vi "Main.vi"() -> ()   [LabVIEW 2017, in "SSH.lvlib"]
doc: "This template is based off of the Queued Message Handler design pattern and the Queued Message Handler project template that ships with LabVIEW.\n\nThe main difference is that the queue is private to this module and communication between modules is performed via Broadcast and Request events.\n\nRequest events are wrapped in public API methods and are handled in the Event Handling Loop (EHL) of this VI. Any module can register for Broadcast events sent by this module. The EHL generates messages based on user interface actions.\n\nThe Message Handling Loop (MHL) processes messages generated by the EHL, or by other messages. The messages are string values, so new messages can be added easily to the Message Cases case structure in the MHL. Each message cluster can also provide an optional value for Message Data, which is a variant that can be converted to whatever message-specific data is required.\n_____\nBased on Delacor QMH Project Template 4.2.1.64."
uses:
  SSH.lvlib
  <vilib>/Delacor/Delacor QMH/Libraries/Cloneable Module Admin_class/Delacor_lib_QMH_Cloneable Module Admin.lvclass
  C:/Program Files (x86)/National Instruments/LabVIEW 2017/vi.lib/Delacor/Delacor QMH/Libraries/Module Admin_class/Delacor_lib_QMH_Module Admin.lvclass
  Connection Info.ctl
  Response Configuration.ctl
  Return Request Configuration.ctl
  Module Data--cluster.ctl
  <vilib>/Delacor/Delacor QMH/Libraries/Cloneable Module Admin_class/Delacor_lib_QMH_Cloneable Module Admin.lvclass/Delacor_lib_QMH_Cloneable Module Admin.ctl
  <vilib>/Delacor/Delacor QMH/Libraries/Message Queue_class/Delacor_lib_QMH_Message Queue.lvclass/Delacor_lib_QMH_Message Queue.ctl
  Stop Argument--cluster.ctl
  <vilib>/Delacor/Delacor QMH/Libraries/Module Admin_class/Delacor_lib_QMH_Module Admin.lvclass/Delacor_lib_QMH_Module Admin.ctl
  Write Command Argument--cluster.ctl
  Write Command (Reply Payload)--cluster.ctl
  Set Response Configuration Argument--cluster.ctl
  <vilib>/Delacor/Delacor QMH/Libraries/Cloneable Module Admin_class/Delacor_lib_QMH_Get Module ID.vi
  <vilib>/Delacor/Delacor QMH/Libraries/Message Queue_class/Delacor_lib_QMH_Enqueue Message (Single).vi
  <vilib>/Delacor/Delacor QMH/Libraries/Module Admin_class/Delacor_lib_QMH_Get External Launch.vi
  <vilib>/Utility/error.llb/Error Cluster From Error Code.vi
  C:/Users/ukhornp/Documents/SSH/References/Renci.SshNet.dll
  References/Renci.SshNet.dll
  <vilib>/ErrorRing/Error Ring.xnode
  <vilib>/Delacor/Delacor QMH/Libraries/Message Queue_class/Delacor_lib_QMH_Message Queue.lvclass
  Clone Registration/Clone Registration.lvlib
panel:
  in  "Response Configuration":T1
  out "Output":string
  out "Return Payload":string
  in  "Command":string
  in  "Connection Info":T2={"host IP"="", "port"=22, "username"="lanforge", "password"="lanforge", "Connection Name"=""}
  in  "Simulate MHL Error":bool
  in  "Simulate EHL Error":bool
  out "error out":errorcluster
  in  "Module Admin":refnum<class "Delacor_lib_QMH_Cloneable Module Admin.lvclass">
  out "Status":string
  # "Other QMH Modules communicate with this Module via its Public API (wrappers for its Request Events).\n\nThis Module communicates with other Modules via its Broadcast Events.\nAny module that wants to get these messages, just registers for this module's Broadcast events."
  # "This template is for the Delacor Modified Queued Message Handler design pattern.\n\nSee the block diagram for more information on how to use this template."
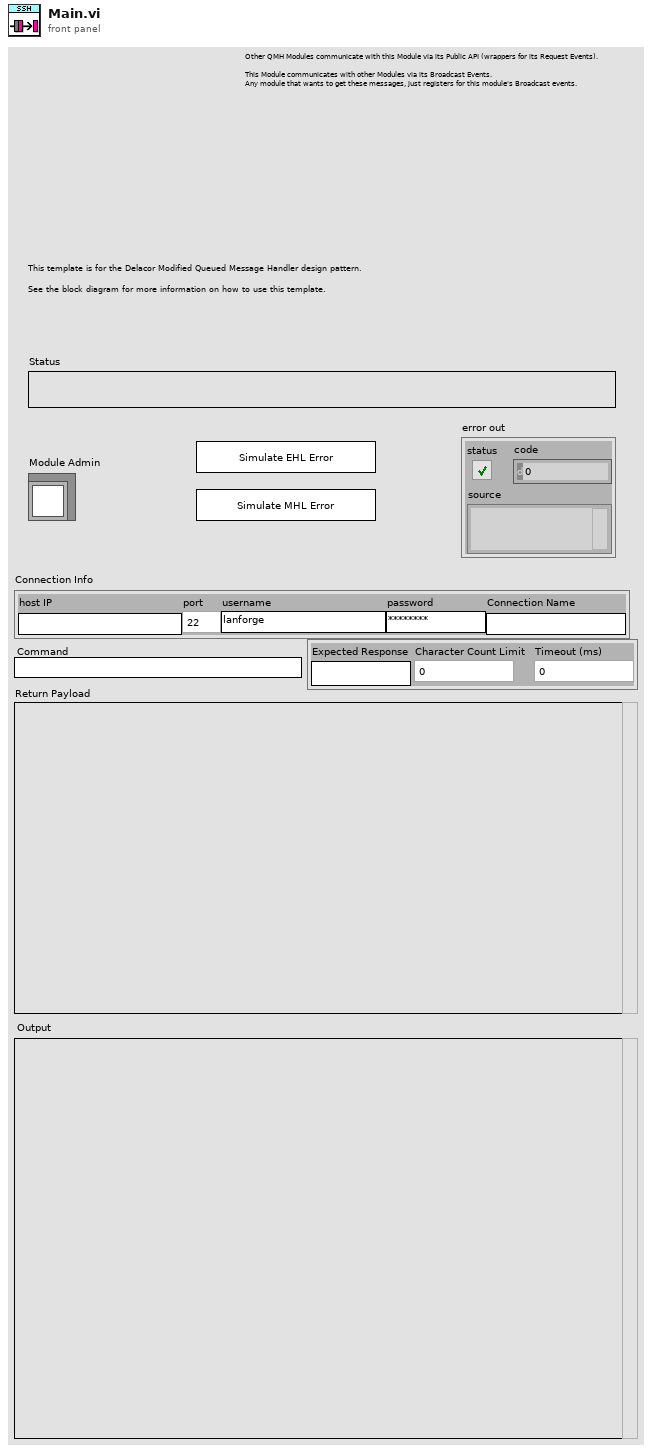
[diagram p1: front panel]
types:
  T1 = typedef "SSH.lvlib/Response Configuration.ctl" = cluster{"Expected Response":string, "Character Count Limit":i32, "Timeout (ms)":u32}
  T2 = typedef "SSH.lvlib/Connection Info.ctl" = cluster{"host IP":string, "port":i32, "username":string, "password":string, "Connection Name":string}
  T3 = typedef "SSH.lvlib/Return Request Configuration.ctl" = cluster{"Response Configuration":T1, "Return Notifier":refnum<notifier>, "Response Requested":bool, "Command":string, "Initial Timer Value":u32}
  T4 = typedef "SSH.lvlib/Request Events--cluster.ctl" = cluster{"Stop Module":refnum<user-event>, "Show Panel":refnum<user-event>, "Hide Panel":refnum<user-event>, "Show Diagram":refnum<user-event>, "Get Module Execution Status":refnum<user-event>, "Write Command":refnum<user-event>, "Set Response Configuration":refnum<user-event>}
  T5 = typedef "SSH.lvlib/Module Data--cluster.ctl" = cluster{"Status":string, "SSH Client Reference":refnum<k24>, "Shell Stream Reference":refnum<k24>, "Stream Writer Reference":refnum<k24>, "Response Configuration":T1}
  T6 = enum32{"invalid lock state", "Not Locked", "Locked (No Password)", "Password-protected"}
  T7 = typedef "SSH.lvlib/Stop Argument--cluster.ctl" = cluster{"Module ID":i32, "Origin":string, "Exit via Stop Module Req?":bool, "Wait for Module to stop?":bool}
  T8 = typedef "SSH.lvlib/Write Command Argument--cluster.ctl" = cluster{"Module ID":i32, "Command":string, "Wait Notifier":refnum<notifier>, "wait for reply":bool}
  T9 = typedef "SSH.lvlib/Set Response Configuration Argument--cluster.ctl" = cluster{"Module ID":i32, "Response Configuration":T1}
  T10 = enum32{"Invalid", "Standard", "Closed", "Hidden", "Minimized", "Maximized"}
  T11 = typedef "SSH.lvlib/dotNET references.ctl" = cluster{"SSH Client Reference":refnum<k24>, "Shell Stream Reference":refnum<k24>}
  T12 = typedef "eventvkey.ctl" = enum16{"ASCII", "Enter", "Return", "Shift", "Ctrl", "Alt", "Cmd", "Opt", "Caps", "NumLock", "Clear", "Break", "Up", "Down", "Left", "Right", "Insert", "Delete", "Home", "End", "PageUp", "PageDown", "Escape", "Help", "Pause", "ScrollLock", "F1", "F2", "F3", "F4", "F5", "F6", "F7", "F8", "F9", "F10", "F11", "F12", "F13", "F14", "F15", "F16", "F17", "F18", "F19", "F20", "F21", "F22", "F23", "F24", "Play", "VolumeUp", "VolumeDown", "Mute", "Two Byte Char"}
  T13 = typedef "SSH.lvlib/Write Command (Reply Payload)--cluster.ctl" = cluster{"Write Command_error":errorcluster, "Return String Payload":string}
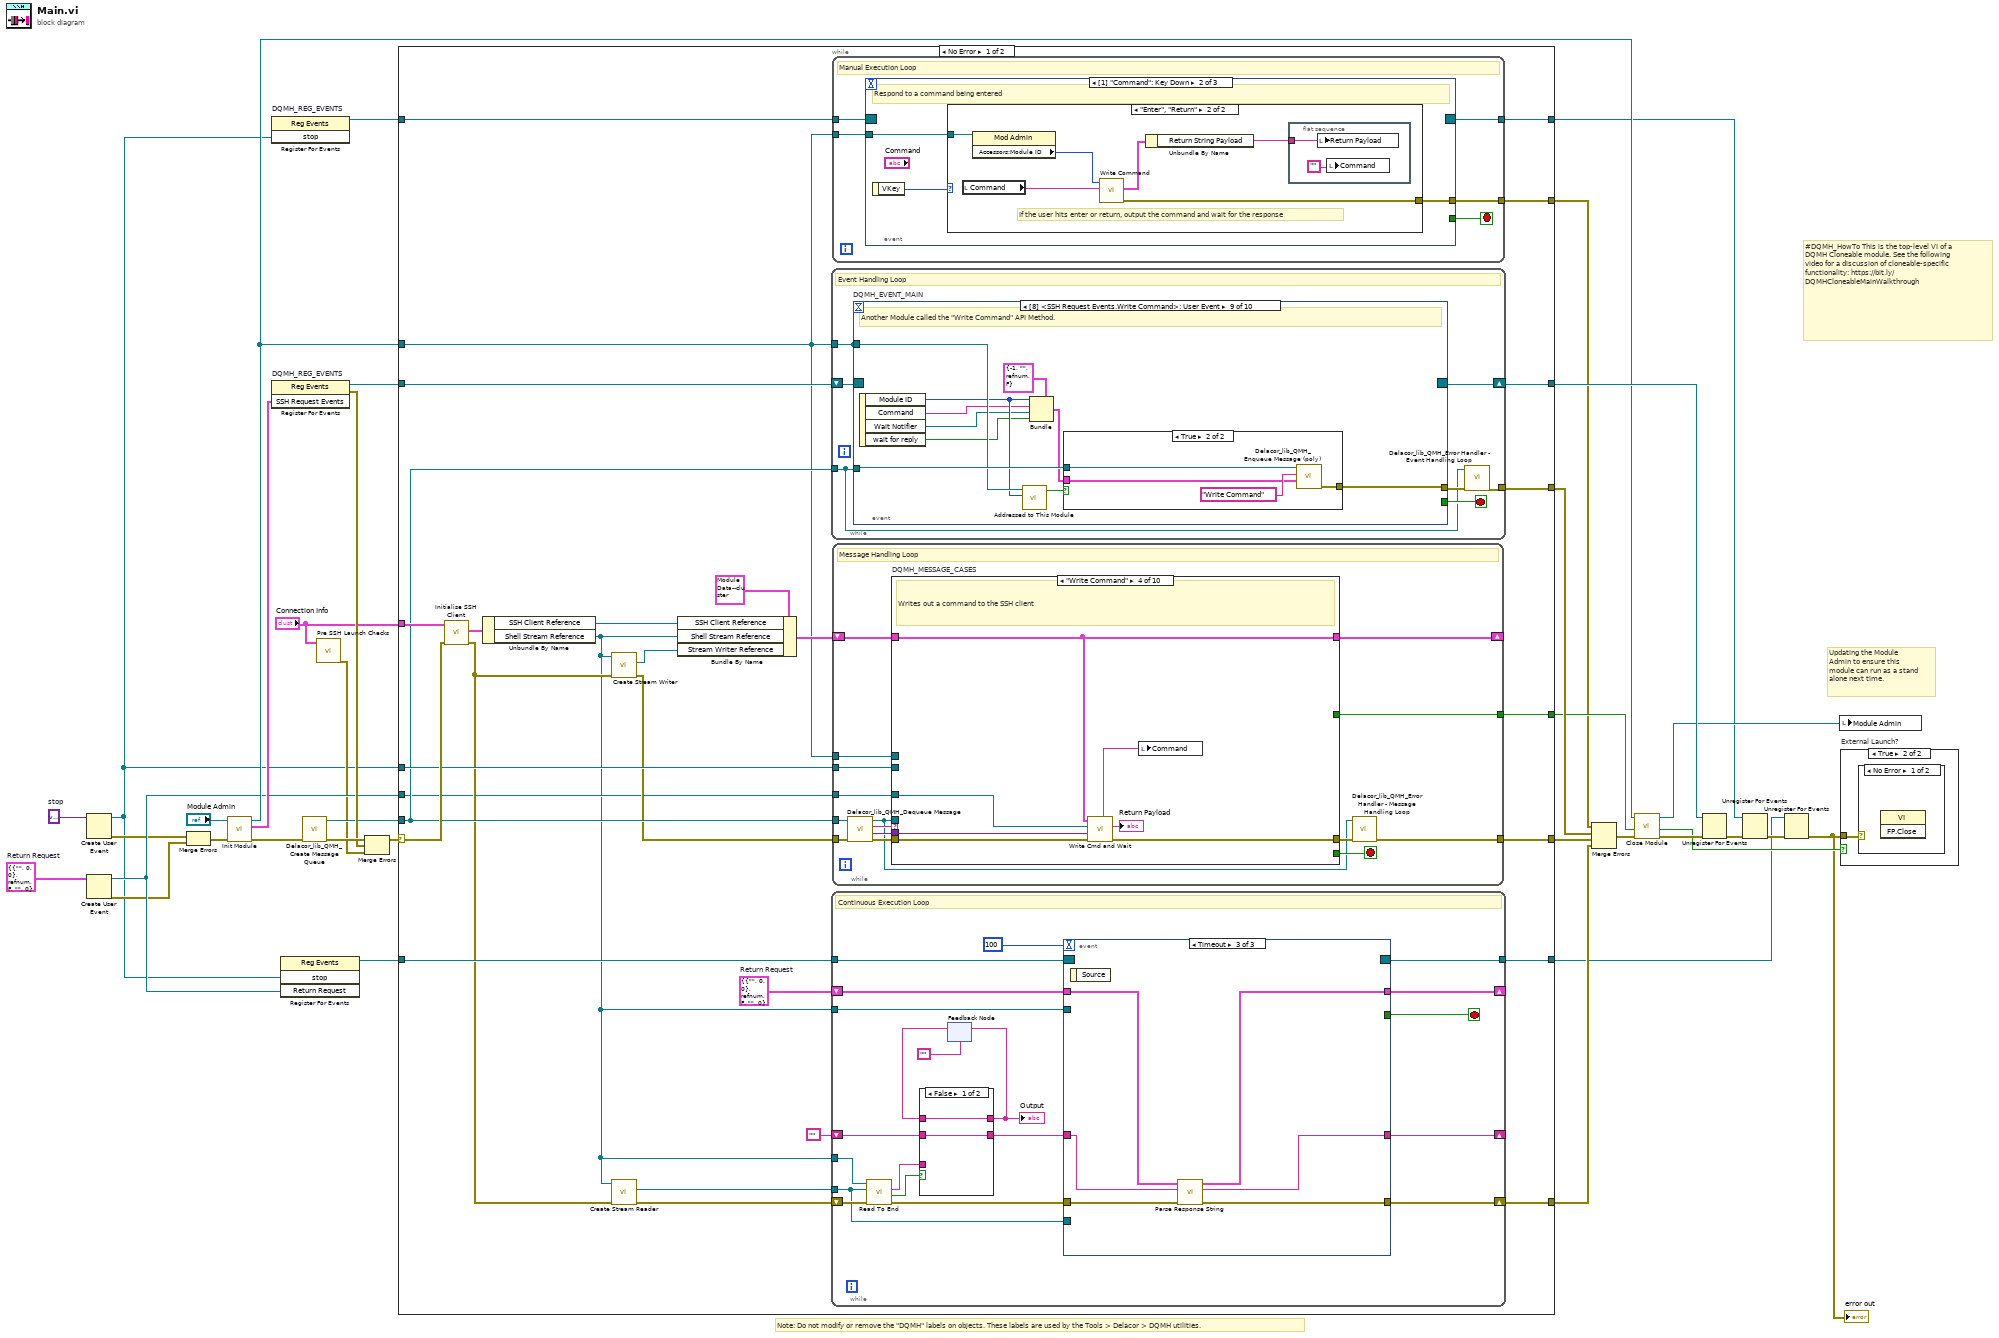
[diagram p0: block diagram]
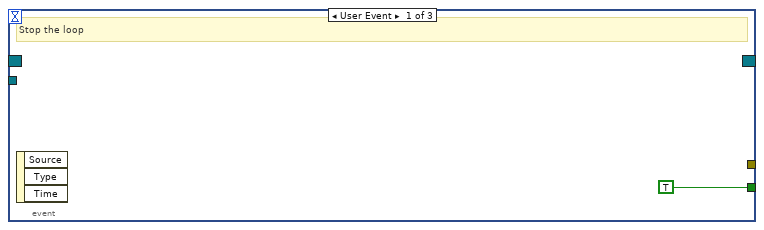
[diagram p2: hidden frame]
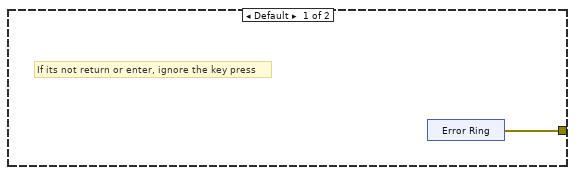
[diagram p3: hidden frame]
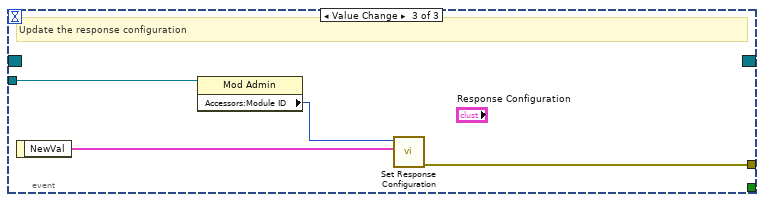
[diagram p4: hidden frame]
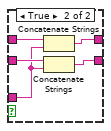
[diagram p5: hidden frame]
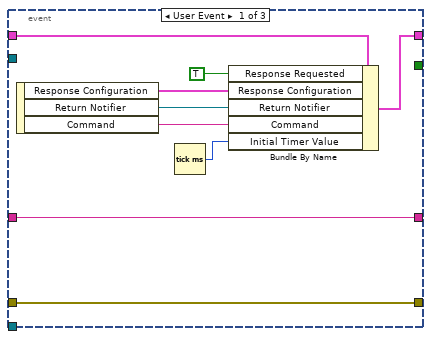
[diagram p6: hidden frame]
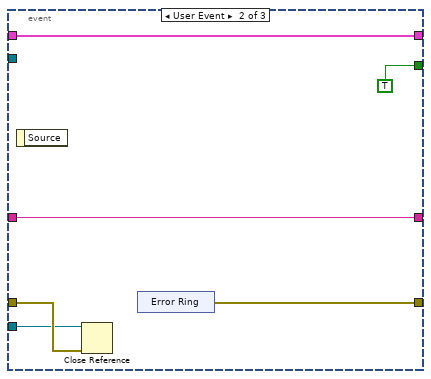
[diagram p7: hidden frame]
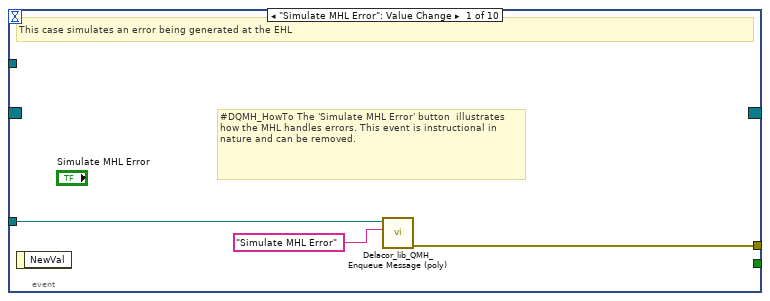
[diagram p8: hidden frame]
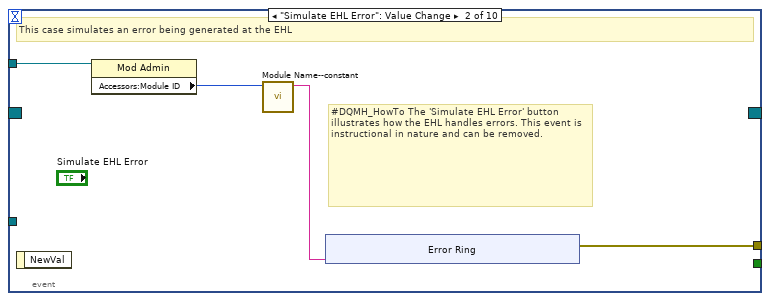
[diagram p9: hidden frame]
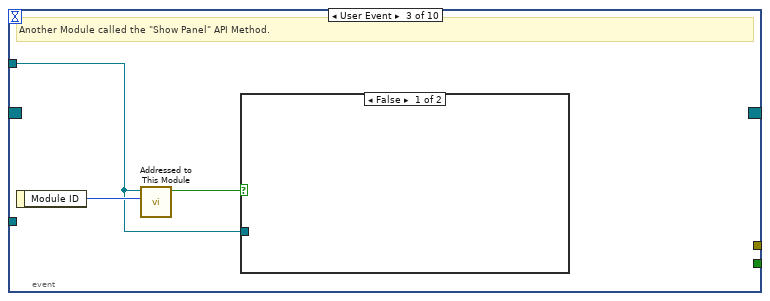
[diagram p10: hidden frame]
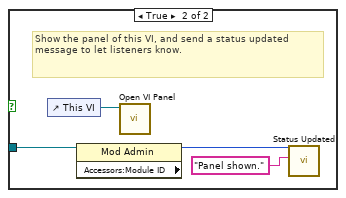
[diagram p11: hidden frame]
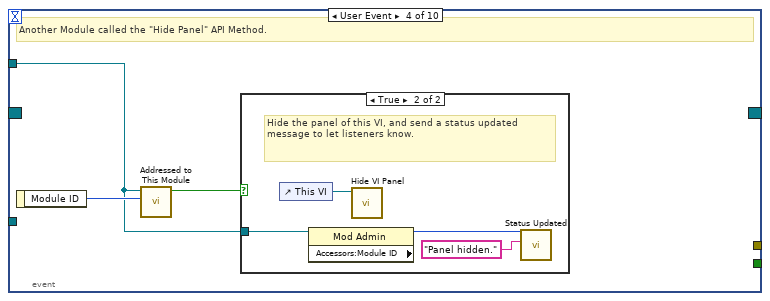
[diagram p12: hidden frame]
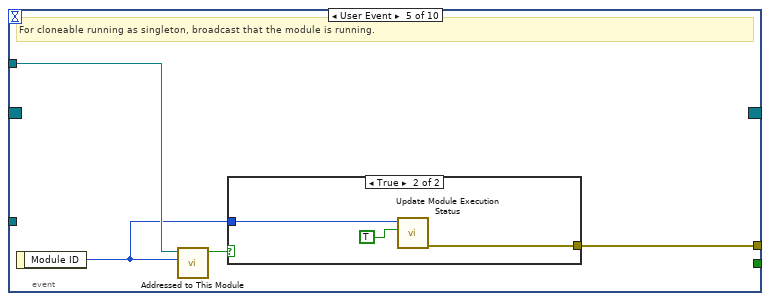
[diagram p14: hidden frame]
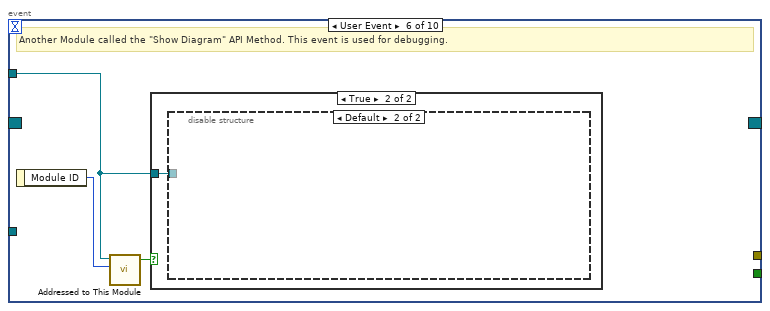
[diagram p16: hidden frame]
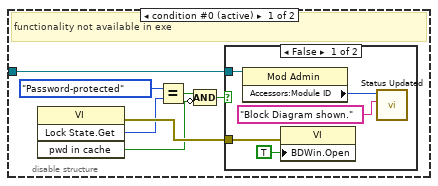
[diagram p18: hidden frame]
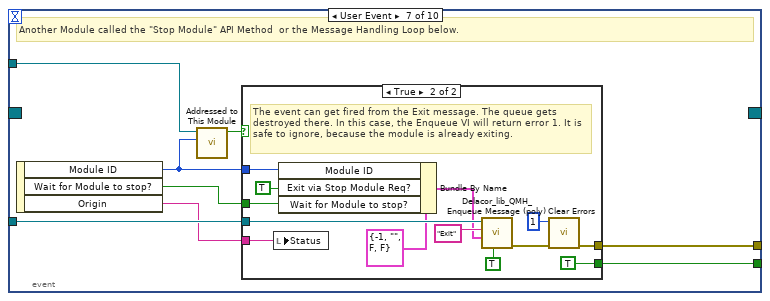
[diagram p20: hidden frame]
diagram:
  w14 = T3 {"Response Configuration"={"Expected Response"="", "Character Count Limit"=0, "Timeout (ms)"=0}, "Return Notifier"=refnum, "Response Requested"=FALSE, "Command"="", "Initial Timer Value"=0}  # Return Request
  w17 = variant  # stop
  # "#DQMH_HowTo This is the top-level VI of a DQMH Cloneable module. See the following video for a discussion of cloneable-specific functionality: https://bit.ly/DQMHCloneableMainWalkthrough"
  # "Note: Do not modify or remove the \"DQMH\" labels on objects. These labels are used by the Tools > Delacor > DQMH utilities."
  # "Updating the Module Admin to ensure this module can run as a stand alone next time."
  n1 = Create User Event(user event datatype=w17) -> (user event=w5:refnum<user-event>, error out=w10:errorcluster)  [unwired: 1 in]
  n2 = Create User Event(user event datatype=w14) -> (user event=w13:refnum<user-event>, error out=w11:errorcluster)  [unwired: 1 in]
  n3 = Merge Errors(w10, w11) -> (w9:errorcluster)
  n4 = call "Init Module.vi"("error in (no error)"=w9, "Cloneable Module Admin in"="Module Admin") -> ("error out"=w32:errorcluster, "SSH Request Events"=w24:T4, "Cloneable Module Admin out"=w21:refnum<class "Delacor_lib_QMH_Cloneable Module Admin.lvclass">)  [unwired: 7 in]
  n5 = register-events "DQMH_REG_EVENTS"(w5) -> (reference out=w6:refnum<event-registration>)  [unwired: 2 in, 1 out]
  n6 = register-events "DQMH_REG_EVENTS"(w24) -> (reference out=w25:refnum<event-registration>, error out=w27:errorcluster)  [unwired: 2 in]
  n7 = register-events(w5, w13) -> (reference out=w16:refnum<event-registration>)  [unwired: 2 in, 1 out]
  n8 = call <vilib>:"Delacor_lib_QMH_Create Message Queue.vi"("error in (no error)"=w32) -> ("error out"=w29:errorcluster, "Message Queue"=w23:refnum<class "Delacor_lib_QMH_Message Queue.lvclass">)  [unwired: 9 in]
  n9 = call "Pre SSH Launch Checks.vi"("Connection Info"="Connection Info") -> ("error out"=w7:errorcluster)  [unwired: 10 in]
  n10 = Merge Errors(w29, w27, w7) -> (w28:errorcluster)
  n11 = case shown="No Error" w28 {
    selector: w28 -> [w57 w387]
    tunnel: [w64 w387] -> w33
    tunnel: [w62 w386] -> w26
    tunnel: w25 -> [w60 w386]
    tunnel: w23 -> [w50 _]
    tunnel: [w63 _] -> w34
    tunnel: w21 -> [w38 w382]
    tunnel: [w59 _] -> w19
    tunnel: "Connection Info" -> [w56 _]
    tunnel: [w53 w379] -> w1
    tunnel: w16 -> [w52 w379]
    tunnel: w5 -> [w51 _]
    tunnel: w13 -> [w44 _]
    tunnel: [w43 _] -> w12
    tunnel: w6 -> [w39 w378]
    tunnel: [w37 _] -> w4
    tunnel: [w36 w378] -> w2
    frame No Error {
      w42 = T3 {"Response Configuration"={"Expected Response"="", "Character Count Limit"=0, "Timeout (ms)"=0}, "Return Notifier"=refnum, "Response Requested"=FALSE, "Command"="", "Initial Timer Value"=0}  # Return Request
      n12 = call "Initialise SSH Client.vi"("error in (no error)"=w57, "Connection Info"=w56) -> ("error out"=w47:errorcluster, "References"=w55:T11)  [unwired: 8 in]
      n13 = Unbundle By Name(w55) -> ("SSH Client Reference"=w54:refnum<k24>, "Shell Stream Reference"=w41:refnum<k24>)
      n14 = call "Create Stream Writer.vi"("error in (no error)"=w47, "Shell Stream Ref"=w41) -> ("error out"=w48:errorcluster, "Stream Writer ref"=w49:refnum<k24>)  [unwired: 8 in]
      n15 = call "Create Stream Reader.vi"("error in (no error)"=w47, "Shell Stream Ref"=w41) -> ("error out"=w46:errorcluster, "Stream Reader Ref"=w45:refnum<k24>)  [unwired: 8 in]
      n16 = Bundle By Name(cluster=T5 {"Status"="", "SSH Client Reference"=refnum, "Shell Stream Reference"=refnum, "Stream Writer Reference"=refnum, "Response Configuration"={"Expected Response"="", "Character Count Limit"=0, "Timeout (ms)"=0}} ("Data Cluster"), "SSH Client Reference"=w54, "Shell Stream Reference"=w41, "Stream Writer Reference"=w49) -> (w58:T5)
      n17 = while {
        tunnel: w50 -> [w138]
        shift-right: [w140] -> w62
        shift-left: w60 -> [w141]
        tunnel: [w142] -> w63
        tunnel: w38 -> [w137]
        tunnel: [w137] -> _
        stop <- w139 stop-if-true
        # "Event Handling Loop"
        n18 = event "DQMH_EVENT_MAIN" shown="[8] <SSH Request Events.Write Command>: User Event" {
          selector: w141 -> [_ _ _ _ _ _ _ _ _ _]
          dyn-events: [_ _ _ _ _ _ _ _ _ _] -> w140
          timeout: _ -> [_ _ _ _ _ _ _ _ _ _]
          tunnel: [_ _ _ _ _ _ w198 _ _ _] -> w139
          tunnel: w138 -> [w145 _ _ _ _ _ w201 w217 w235 w247]
          tunnel: [w146 w150 _ _ w175 _ w202 w220 w228 w240] -> w143
          tunnel: w137 -> [_ w149 w158 w165 w173 w179 w200 w218 w233 w245]
          event "Simulate MHL Error": Value Change {
            # "#DQMH_HowTo The 'Simulate MHL Error' button  illustrates how the MHL handles errors. This event is instructional in nature and can be removed."
            # "This case simulates an error being generated at the EHL"
            n19 = event-data() -> ()  [unwired: 1 in, 1 out]
            n20 = call-poly <vilib>:"Delacor_lib_QMH_Enqueue Message (poly).vi"("Message"="Simulate MHL Error", "Message Queue in"=w145) -> ("error out"=w146:errorcluster)  [unwired: 8 in, 1 out]
          }
          event "Simulate EHL Error": Value Change {
            # "#DQMH_HowTo The 'Simulate EHL Error' button  illustrates how the EHL handles errors. This event is instructional in nature and can be removed."
            # "This case simulates an error being generated at the EHL"
            n21 = event-data() -> ()  [unwired: 1 in, 1 out]
            n22 = property class="Mod Admin"(reference=w149) -> ("Accessors:Module ID"=w148:i32)  [unwired: 1 in, 2 out]
            n23 = call "Module Name--constant.vi"("Module ID"=w148) -> ("Module Name"=w147:string)  [unwired: 10 in]
            n24 = xnode "Error Ring"("parameter 0"=w147) -> ("error out"=w150:errorcluster)
          }
          event User Event {
            # "Another Module called the \"Show Panel\" API Method."
            n25 = event-data() -> ("Module ID"=w159:i32)  [unwired: 1 in]
            n26 = call "Addressed to This Module.vi"("Module ID from Argument"=w159, "Module Admin"=w158) -> ("Addressed to this instance?"=w160:bool)  [unwired: 8 in, 1 out]
            n27 = case shown="False" w160 {
              tunnel: w158 -> [_ w162]
              frame False {
              }
              frame True {
                # "Show the panel of this VI, and send a status updated message to let listeners know."
                n28 = control-ref of="This VI"() -> (w164:refnum<vi>)
                n29 = property class="Mod Admin"(reference=w162) -> ("Accessors:Module ID"=w161:i32)  [unwired: 1 in, 2 out]
                n30 = call "Open VI Panel.vi"("VI"=w164) -> ()  [unwired: 10 in, 1 out]
                n31 = call "Status Updated.vi"("Status"="Panel shown." ("format string"), "Module ID"=w161) -> ()  [unwired: 9 in, 1 out]
              }
            }
          }
          event User Event {
            # "Another Module called the \"Hide Panel\" API Method."
            n32 = event-data() -> ("Module ID"=w166:i32)  [unwired: 1 in]
            n33 = call "Addressed to This Module.vi"("Module ID from Argument"=w166, "Module Admin"=w165) -> ("Addressed to this instance?"=w167:bool)  [unwired: 8 in, 1 out]
            n34 = case shown="True" w167 {
              tunnel: w165 -> [_ w169]
              frame False {
              }
              frame True {
                # "Hide the panel of this VI, and send a status updated message to let listeners know."
                n35 = control-ref of="This VI"() -> (w171:refnum<vi>)
                n36 = property class="Mod Admin"(reference=w169) -> ("Accessors:Module ID"=w168:i32)  [unwired: 1 in, 2 out]
                n37 = call "Hide VI Panel.vi"("VI"=w171) -> ()  [unwired: 10 in, 1 out]
                n38 = call "Status Updated.vi"("Status"="Panel hidden." ("format string"), "Module ID"=w168) -> ()  [unwired: 9 in, 1 out]
              }
            }
          }
          event User Event {
            # "For cloneable running as singleton, broadcast that the module is running."
            n39 = event-data() -> ("Module ID"=w172:i32)  [unwired: 1 in]
            n40 = call "Addressed to This Module.vi"("Module ID from Argument"=w172, "Module Admin"=w173) -> ("Addressed to this instance?"=w174:bool)  [unwired: 8 in, 1 out]
            n41 = case shown="True" w174 {
              tunnel: [_ w178] -> w175
              tunnel: w172 -> [_ w177]
              frame False {
              }
              frame True {
                n42 = call "Update Module Execution Status.vi"("Running?"=TRUE, "Module ID"=w177) -> ("error out"=w178:errorcluster)  [unwired: 9 in]
              }
            }
          }
          event User Event {
            # "Another Module called the \"Show Diagram\" API Method. This event is used for debugging."
            n43 = event-data() -> ("Module ID"=w180:i32)  [unwired: 1 in]
            n44 = call "Addressed to This Module.vi"("Module ID from Argument"=w180, "Module Admin"=w179) -> ("Addressed to this instance?"=w181:bool)  [unwired: 8 in, 1 out]
            n45 = case shown="True" w181 {
              tunnel: w179 -> [_ w182]
              frame False {
              }
              frame True {
                n46 = disable-structure shown="Default" {
                  disable-tunnel: w182 -> [w183 _]
                  frame condition #0 (active) {
                    # "functionality not available in exe"
                    n47 = invoke class="VI" method="Lock State.Get"() -> (error out=w189:errorcluster, "Get Lock State"=w188:T6, "pwd in cache"=w185:bool)  [unwired: 4 in, 1 out]
                    n48 = Equal?(x=T6."Password-protected", y=w188) -> (x = y?=w186:bool)
                    n49 = Compound Arithmetic op=AND(w186, invert w185) -> (w184:bool)
                    n50 = case shown="False" w184 {
                      tunnel: w189 -> [w194 _]
                      tunnel: w183 -> [w191 _]
                      frame False {
                        n51 = property class="Mod Admin"(reference=w191) -> ("Accessors:Module ID"=w190:i32)  [unwired: 1 in, 2 out]
                        n52 = property class="VI"(error in=w194, "BDWin.Open"=TRUE ("Block Diagram Window:Open")) -> ()  [unwired: 1 in, 2 out]
                        n53 = call "Status Updated.vi"("Status"="Block Diagram shown." ("format string"), "Module ID"=w190) -> ()  [unwired: 9 in, 1 out]
                      }
                      frame True {
                        # "Password-protected VI, and the password is not in the cache. Do not show the diagram."
                      }
                    }
                  }
                  frame condition #1 {
                  }
                }
              }
            }
          }
          event User Event {
            # "Another Module called the \"Stop Module\" API Method  or the Message Handling Loop below."
            n54 = event-data() -> ("Module ID"=w196:i32, "Wait for Module to stop?"=w197:bool, "Origin"=w195:string)  [unwired: 1 in]
            n55 = call "Addressed to This Module.vi"("Module ID from Argument"=w196, "Module Admin"=w200) -> ("Addressed to this instance?"=w199:bool)  [unwired: 8 in, 1 out]
            n56 = case shown="True" w199 {
              tunnel: [_ w214] -> w202
              tunnel: w201 -> [_ w210]
              tunnel: [_ TRUE] -> w198
              tunnel: w197 -> [_ w205]
              tunnel: w196 -> [_ w207]
              tunnel: w195 -> [_ w203]
              frame False {
              }
              frame True {
                # "The event can get fired from the Exit message. The queue gets destroyed there. In this case, the Enqueue VI will return error 1. It is safe to ignore, because the module is already exiting."
                n57 = local write "Status"(w203) -> ()
                n58 = Bundle By Name(cluster=T7 {"Module ID"=-1, "Origin"="", "Exit via Stop Module Req?"=FALSE, "Wait for Module to stop?"=FALSE} ("Stop Argument"), "Module ID"=w207, "Exit via Stop Module Req?"=TRUE, "Wait for Module to stop?"=w205) -> (w204:T7)
                n59 = call-poly <vilib>:"Delacor_lib_QMH_Enqueue Message (poly).vi"("Priority Message? (F)"=TRUE, "Message Data"=w204, "Message"="Exit", "Message Queue in"=w210) -> ("error out"=w215:errorcluster)  [unwired: 6 in, 1 out]
                n60 = call <vilib>:"Clear Errors.vi"("error in (no error)"=w215, "specific error code to clear (0: all)"=1) -> ("error out"=w214:errorcluster)  [unwired: 4 in, 1 out]
              }
            }
          }
          event Panel Close? {
            w219 = TRUE  # Discard the event, the MHL is responsible for closing and stopping this VI.
            # "Hide the panel or send the 'Exit' message if the user clicks the 'X' on the module main VI panel."
            n61 = event-data() -> ()  [unwired: 1 in, 1 out]
            n62 = property class="Mod Admin"(reference=w218) -> ("Accessors:External Launch"=w216:bool)  [unwired: 1 in, 2 out]
            n63 = case shown="True" w216 {
              tunnel: w217 -> [_ w224]
              tunnel: [_ w225] -> w220
              frame True {
                # "If externally launched, clicking the 'X' hides the panel, but doesn't close it."
                n64 = control-ref of="This VI"() -> (w221:refnum<vi>)
                n65 = call "Hide VI Panel.vi"("VI"=w221) -> ()  [unwired: 10 in, 1 out]
              }
              frame False {
                # "If run as a stand-alone VI, clicking the panel 'X' stops the VI."
                n66 = call-poly <vilib>:"Delacor_lib_QMH_Enqueue Message (poly).vi"("Priority Message? (F)"=TRUE, "Message"="Exit", "Message Queue in"=w224) -> ("error out"=w225:errorcluster)  [unwired: 7 in, 1 out]
              }
            }
            n67 = event-data("Discard?"=w219) -> ()  [unwired: 1 in, 1 out]
          }
          event User Event {
            # "Another Module called the \"Write Command\" API Method."
            n68 = event-data() -> ("Module ID"=w230:i32, "Command"=w229:string, "Wait Notifier"=w227:refnum<notifier>, "wait for reply"=w226:bool)  [unwired: 1 in]
            n69 = call "Addressed to This Module.vi"("Module ID from Argument"=w230, "Module Admin"=w233) -> ("Addressed to this instance?"=w234:bool)  [unwired: 8 in, 1 out]
            n70 = Bundle(cluster=T8 {"Module ID"=-1, "Command"="", "Wait Notifier"=refnum, "wait for reply"=FALSE} ("Write Command Argument"), "Module ID"=w230, "Command"=w229, "Wait Notifier"=w227, "wait for reply"=w226) -> (w231:T8)
            n71 = case shown="True" w234 {
              tunnel: w235 -> [_ w239]
              tunnel: w231 -> [_ w237]
              tunnel: [_ w236] -> w228
              frame False {
              }
              frame True {
                n72 = call-poly <vilib>:"Delacor_lib_QMH_Enqueue Message (poly).vi"("Message Data"=w237, "Message"="Write Command", "Message Queue in"=w239) -> ("error out"=w236:errorcluster)  [unwired: 7 in, 1 out]
              }
            }
          }
          event User Event {
            # "Another Module called the \"Set Return String\" API Method."
            n73 = event-data() -> ("Module ID"=w242:i32, "Response Configuration"=w241:T1)  [unwired: 1 in]
            n74 = Bundle(cluster=T9 {"Module ID"=-1, "Response Configuration"={"Expected Response"="", "Character Count Limit"=0, "Timeout (ms)"=0}} ("Set Return String Argument"), "Module ID"=w242, "Response Configuration"=w241) -> (w243:T9)
            n75 = call "Addressed to This Module.vi"("Module ID from Argument"=w242, "Module Admin"=w245) -> ("Addressed to this instance?"=w246:bool)  [unwired: 8 in, 1 out]
            n76 = case shown="True" w246 {
              tunnel: w247 -> [_ w251]
              tunnel: w243 -> [_ w249]
              tunnel: [_ w248] -> w240
              frame False {
              }
              frame True {
                n77 = call-poly <vilib>:"Delacor_lib_QMH_Enqueue Message (poly).vi"("Message Data"=w249, "Message"="Set Response Configuration", "Message Queue in"=w251) -> ("error out"=w248:errorcluster)  [unwired: 7 in, 1 out]
              }
            }
          }
        }
        n78 = call-dynamic "Delacor_lib_QMH_Error Handler - Event Handling Loop.vi"("error in (no error)"=w143, "Message Queue in"=w138) -> ("dup error in"=w142:errorcluster)  [unwired: 8 in, 1 out]
      }
      n79 = while {
        tunnel: [w107] -> w53
        tunnel: w52 -> [w106]
        tunnel: w45 -> [w97]
        tunnel: w41 -> [w103]
        shift-right: [w100] -> w43
        shift-left: w46 -> [w104]
        shift-right: [w102] -> _
        shift-left: w42 -> [w101]
        tunnel: w41 -> [w96]
        shift-right: [w91] -> _
        shift-left: "" -> [w93]
        stop <- w105 stop-if-true
        # "Continuous Execution Loop"
        n80 = call "Read To End.vi"("error in (no error)"=w104, "Stream Reader Ref"=w97, "Shell Stream Reference"=w96) -> ("error out"=w98:errorcluster, "DataAvailable"=w95:bool, "ReadToEnd"=w94:string)  [unwired: 6 in]
        n81 = feedback #1("") -> (w90:string)
        n82 = case shown="False" w95 {
          tunnel: w94 -> [_ w111]
          tunnel: w90 -> [w109 w114]
          tunnel: [w109 w113] -> w88
          tunnel: w93 -> [w108 w112]
          tunnel: [w108 w110] -> w92
          frame False {
          }
          frame True {
            n83 = Concatenate Strings(w114, w111) -> (w113:string)
            n84 = Concatenate Strings(w112, w111) -> (w110:string)
          }
        }
        "Output" <- w88
        n85 = feedback-in #1(w88) -> ()
        n86 = event shown="[2] Timeout" {
          selector: w106 -> [_ _ _]
          dyn-events: [_ _ _] -> w107
          timeout: 100 -> [_ _ _]
          tunnel: [_ TRUE _] -> w105
          tunnel: w97 -> [_ w127 _]
          tunnel: w98 -> [w123 w128 w136]
          tunnel: w103 -> [_ _ _]
          tunnel: [w123 w126 w135] -> w100
          tunnel: [w120 w125 w133] -> w102
          tunnel: w101 -> [w119 w125 w134]
          tunnel: w92 -> [w117 w124 w132]
          tunnel: [w117 w124 w131] -> w91
          event User Event {
            n87 = event-data() -> ("Response Configuration"=w121:T1, "Return Notifier"=w122:refnum<notifier>, "Command"=w115:string)  [unwired: 1 in]
            n88 = Tick Count (ms)() -> (millisecond timer value=w116:u32)
            n89 = Bundle By Name(cluster=w119, "Response Requested"=TRUE, "Response Configuration"=w121, "Return Notifier"=w122, "Command"=w115, "Initial Timer Value"=w116) -> (w120:T3)
          }
          event User Event {
            n90 = event-data() -> ()  [unwired: 1 in, 1 out]
            n91 = Close Reference(reference=w127, error in (no error)=w128) -> ()  [unwired: 1 out]
            n92 = xnode "Error Ring"() -> ("error out"=w126:errorcluster)
          }
          event Timeout {
            n93 = event-data() -> ()  [unwired: 1 in, 1 out]
            n94 = call "Parse Response String.vi"("error in (no error)"=w136, "Response String in"=w132, "Return Request in"=w134) -> ("error out"=w135:errorcluster, "Response String out"=w131:string, "Return Request out"=w133:T3)  [unwired: 6 in]
          }
        }
      }
      n95 = while {
        tunnel: w39 -> [w69]
        tunnel: w38 -> [w67]
        tunnel: [w66] -> w37
        tunnel: [w65] -> w36
        stop <- w68 stop-if-true
        # "Manual Execution Loop"
        n96 = event shown="[1] \"Command\": Key Down" {
          selector: w69 -> [_ _ _]
          dyn-events: [_ _ _] -> w65
          timeout: _ -> [_ _ _]
          tunnel: [TRUE _ _] -> w68
          tunnel: w67 -> [_ w73 w85]
          tunnel: [_ w71 w84] -> w66
          event User Event {
            # "Stop the loop"
            n97 = event-data() -> ()  [unwired: 1 in, 3 out]
          }
          event "Command": Key Down {
            # "Respond to a command being entered"
            n98 = event-data() -> ("VKey"=w72:T12)  [unwired: 1 in]
            n99 = case shown="\"Enter\", \"Return\"" w72 {
              tunnel: w73 -> [_ w81]
              tunnel: [w74 w76] -> w71
              frame Default {
                # "If its not return or enter, ignore the key press"
                n100 = xnode "Error Ring"() -> ("error out"=w74:errorcluster)
              }
              frame "Enter", "Return" {
                # "If the user hits enter or return, output the command and wait for the response"
                n101 = local read "Command"() -> (w79:string)
                n102 = property class="Mod Admin"(reference=w81) -> ("Accessors:Module ID"=w80:i32)  [unwired: 1 in, 2 out]
                n103 = call "Write Command.vi"("Command"=w79, "Module ID"=w80) -> ("error out"=w76:errorcluster, "Reply Payload"=w78:T13)  [unwired: 7 in, 1 out]
                n104 = Unbundle By Name(w78) -> ("Return String Payload"=w77:string)
                n105 = flat-sequence {
                  tunnel: w77 -> [w83]
                  frame #0 {
                    n106 = local write "Return Payload"(w83) -> ()
                    n107 = local write "Command"("") -> ()
                  }
                }
              }
            }
          }
          event Value Change {
            # "Update the response configuration"
            n108 = event-data() -> ("NewVal"=w86:T1)  [unwired: 1 in]
            n109 = property class="Mod Admin"(reference=w85) -> ("Accessors:Module ID"=w87:i32)  [unwired: 1 in, 2 out]
            n110 = call "Set Response Configuration.vi"("Response Configuration"=w86, "Module ID"=w87) -> ("error out"=w84:errorcluster)  [unwired: 9 in]
          }
        }
      }
      n111 = while {
        tunnel: w50 -> [w257]
        shift-right: [w261] -> _
        shift-left: w58 -> [w262]
        tunnel: w48 -> [w265]
        tunnel: [w263] -> w64
        tunnel: w38 -> [w255]
        tunnel: [w254] -> w59
        tunnel: w51 -> [w253]
        tunnel: w44 -> [w252]
        stop <- w260 stop-if-true
        # "Message Handling Loop"
        n112 = call-dynamic "Delacor_lib_QMH_Dequeue Message.vi"("error in (no error)"=w265, "Message Queue in"=w257) -> ("error out"=w264:errorcluster, "Message Data"=w258:variant, "Message"=w259:string, "Message Queue out"=w256:refnum<class "Delacor_lib_QMH_Message Queue.lvclass">)  [unwired: 6 in]
        n113 = case "DQMH_MESSAGE_CASES" shown="\"Write Command\"" w259 {
          selector: w259 -> [_ _ _ _ _ _ _ _ _ w365]
          tunnel: w256 -> [_ _ _ _ _ _ w309 _ w356 _]
          tunnel: w264 -> [w284 w288 w296 w303 w306 w308 w319 w332 w361 w367]
          tunnel: [w282 w288 w294 w302 w305 w308 w315 w331 w358 w368] -> w266
          tunnel: w262 -> [w275 w287 w295 w300 w304 w307 w314 w329 w343 w366]
          tunnel: [w274 w287 w290 w300 w304 w307 w314 w329 w343 w366] -> w261
          tunnel: [_ _ _ _ _ _ _ _ w355 _] -> w260
          tunnel: w258 -> [_ _ w293 w301 _ _ w313 _ w353 _]
          tunnel: w255 -> [w269 _ _ _ _ _ w312 w327 w349 w363]
          tunnel: [_ _ _ _ _ _ _ _ w351 _] -> w254
          tunnel: w253 -> [_ _ _ _ _ _ _ _ w345 _]
          tunnel: w252 -> [_ _ _ w299 _ _ _ _ w340 _]
          frame "Initialize" {
            w267 = "Initial Message" ("Initial Message")
            # "Initialize - Any operation that needs to be done before the module can receive messages. Synchronize Caller Events.vi will inform Start Module.vi that the module has launched and is ready to receive messages. Module Did Init.vi will broadcast that the module initialized."
            n114 = call "Synchronize Caller Events.vi"("error in (no error)"=w284, "Module Admin"=w269) -> ("error out"=w283:errorcluster, "Module Admin out"=w268:refnum<class "Delacor_lib_QMH_Cloneable Module Admin.lvclass">)  [unwired: 8 in]
            n115 = property class="Mod Admin"(reference=w268) -> ("Accessors:Module ID"=w271:i32, "Accessors:External Launch"=w270:bool)  [unwired: 1 in, 2 out]
            n116 = call "Module Name--constant.vi"("Module ID"=w271) -> ("Module Name"=w279:string)  [unwired: 10 in]
            n117 = property class="VI"("Front Panel.Title"=w279) -> (reference out=w281:refnum<vi>, error out=w286:errorcluster)  [unwired: 2 in]
            n118 = Select(t=T10."Hidden" ("State"), s=w270, f=T10."Standard" ("State")) -> (s? t:f=w276:T10)
            n119 = invoke class="VI" method="FP.Open"(reference=w281, error in=w286, "State"=w276) -> (reference out=w280:refnum<vi>, error out=w285:errorcluster)  [unwired: 2 in, 3 out]
            n120 = call "Module Name--constant.vi"("Module ID"=w271) -> ("Module Name"=w272:string)  [unwired: 10 in]
            n121 = Bundle By Name(cluster=w275, "Status"=w267) -> (w274:T5)
            n122 = invoke class="VI" method="FP.Center"(reference=w280, error in=w285) -> ()  [unwired: 1 in, 3 out]
            n123 = call "Module Did Init.vi"("error in (no error)"=w283, "Initialized?"=TRUE, "Origin"=w272, "Module ID"=w271) -> ("error out"=w282:errorcluster)  [unwired: 7 in]
            "Status" <- w267
          }
          frame "--- Module Specific ---" {
            # "Separator -- The following cases handle messages specific to this Module."
          }
          frame "Set Response Configuration" {
            # "Update the front panel control for the response config"
            # "Sets the trigger condition to return a stream on"
            n124 = Variant To Data(error in=w296, type=T9 {"Module ID"=-1, "Response Configuration"={"Expected Response"="", "Character Count Limit"=0, "Timeout (ms)"=0}} ("Set Return String Argument"), Variant=w293) -> (data=w291:T9, error out=w294:errorcluster)
            n125 = Unbundle By Name(w291) -> ("Response Configuration"=w289:T1)
            n126 = local write "Response Configuration"(w289) -> ()
            n127 = Bundle By Name(cluster=w295, "Response Configuration"=w289) -> (w290:T5)
          }
          frame "Write Command" {
            # "Writes out a command to the SSH client"
            n128 = call "Write Cmd and Wait.vi"("error in (no error)"=w303, "Message Data"=w301, "User Event in"=w299, "Data Cluster"=w300) -> ("error out"=w302:errorcluster, "Return Payload"=→"Return Payload":string, "Command"=w297:string)  [unwired: 5 in]
            n129 = local write "Command"(w297) -> ()
          }
          frame "---Copy This Frame---" {
            # "Duplicate this frame when creating new messages.  Change this comment in the duplicated frame to describe this message."
            n130 = Merge Errors(w306) -> (w305:errorcluster)
          }
          frame "--- Exit and Error Handling---" {
            # "Separator - the following cases handle errors and exit messages."
          }
          frame "Error" {
            # "#CodeRecommended - If you ever change the name of this \"Error\" message, you'll need to update the name in the Check Loop Error.vi as well."
            # "#CodeRecommended - If the module is running in standalone mode (External Launch = FALSE), this code will pop up an error dialog and call the 'Exit' message if an error occurs. Add more fine-grained error handling here."
            # "Error - Check the error message data and respond accordingly. This message is sent by the \"Error Handler\" VIs at the end of each loop in this application."
            n131 = property class="Mod Admin"(reference=w312) -> ("Accessors:External Launch"=w310:bool, "Accessors:Module ID"=w311:i32)  [unwired: 1 in, 2 out]
            n132 = Variant To Data(error in=w319, type=errorcluster {"status"=FALSE, "code"=0, "source"=""} ("error constant"), Variant=w313) -> (data=w320:errorcluster, error out=w317:errorcluster)
            n133 = call "Error Reported.vi"("Error"=w320, "Module ID"=w311) -> ()  [unwired: 9 in, 1 out]
            n134 = case shown="False" w310 {
              tunnel: [w325 _] -> w316
              tunnel: w309 -> [w323 _]
              tunnel: w320 -> [w324 _]
              frame False {
                # "If the module is running standalone, then pop up an error dialog and call the \"Exit\" message."
                n135 = call <vilib>:"Simple Error Handler.vi"("error in (no error)"=w324) -> ()  [unwired: 4 in, 5 out]
                n136 = call-poly <vilib>:"Delacor_lib_QMH_Enqueue Message (poly).vi"("Priority Message? (F)"=TRUE, "Message"="Exit", "Message Queue in"=w323) -> ("error out"=w325:errorcluster)  [unwired: 7 in, 1 out]
              }
              frame True {
                # "If the module was launched externally, calling the Error Reported broadcast VI is the only action performed by the \"Error\" message. The module's caller can then process the error appropriately."
              }
            }
            n137 = Merge Errors(w317, w316) -> (w315:errorcluster)
            n138 = local write "error out"(w315) -> ()
          }
          frame "Simulate MHL Error" {
            # "#DQMH_HowTo The 'Simulate MHL Error' button  illustrates how the MHL handles errors. This event is instructional in nature and can be removed."
            # "Simulate an error occurring at the MHL"
            n139 = property class="Mod Admin"(reference=w327) -> ("Accessors:Module ID"=w328:i32)  [unwired: 1 in, 2 out]
            n140 = call "Module Name--constant.vi"("Module ID"=w328) -> ("Module Name"=w326:string)  [unwired: 10 in]
            n141 = xnode "Error Ring"("parameter 0"=w326) -> ("error out"=w330:errorcluster)
            n142 = Merge Errors(w332, w330) -> (w331:errorcluster)
          }
          frame "Exit" {
            w354 = 91  # 91: not all Exit messages will have an argument
            w355 = TRUE  # Stop the VI
            # "Release the message queue reference"
            # "Exit - Exit the application."
            n143 = Generate User Event(user event=w345, event data cluster=variant ("event data")) -> (user event out=w347:refnum<user-event>, error out=w346:errorcluster)  [unwired: 2 in]
            n144 = Destroy User Event(user event=w340) -> ()  [unwired: 1 in, 1 out]
            n145 = Destroy User Event(user event=w347, error in=w346) -> ()  [unwired: 1 out]
            n146 = Variant To Data(error in=w361, type=T7 {"Module ID"=-1, "Origin"="", "Exit via Stop Module Req?"=FALSE, "Wait for Module to stop?"=FALSE} ("Stop Argument"), Variant=w353) -> (data=w350:T7, error out=w357:errorcluster)
            n147 = call <vilib>:"Clear Errors.vi"("error in (no error)"=w357, "specific error code to clear (0: all)"=w354) -> ("error out"=w360:errorcluster)  [unwired: 4 in, 1 out]
            n148 = control-ref of="This VI"() -> (w348:refnum<vi>)
            n149 = call-dynamic "Delacor_lib_QMH_Release Message Queue.vi"("error in (no error)"=w360, "Message Queue"=w356) -> ("error out"=w359:errorcluster)  [unwired: 9 in]
            n150 = call "Handle Exit.vi"("Stop Argument"=w350, "Module Admin in"=w349, "VI reference"=w348) -> ("error out"=w342:errorcluster, "Wait for Stop?"=w351:bool)  [unwired: 7 in]
            n151 = call "Stop SSH Client.vi"("Module Data"=w343) -> ("error out"=w341:errorcluster)  [unwired: 10 in]
            n152 = Merge Errors(w359, w341, w342) -> (w358:errorcluster)
          }
          frame Default {
            # "'Default' case only runs if there is a message that isn't defined in any of the other cases.  Output a programming error."
            n153 = property class="Mod Admin"(reference=w363) -> ("Accessors:Module ID"=w362:i32)  [unwired: 1 in, 2 out]
            n154 = call "Module Name--constant.vi"("Module ID"=w362) -> ("Module Name"=w364:string)  [unwired: 10 in]
            n155 = xnode "Error Ring"("parameter 0"=w365, "parameter 1"=w364) -> ("error out"=w369:errorcluster)
            n156 = Merge Errors(w367, w369) -> (w368:errorcluster)
          }
        }
        n157 = call-dynamic "Delacor_lib_QMH_Error Handler - Message Handling Loop.vi"("error in (no error)"=w266, "Message Queue in"=w256) -> ("dup error in"=w263:errorcluster)  [unwired: 8 in, 1 out]
      }
    }
    frame Error {
      n158 = call "Synchronize Caller Events.vi"("Module Admin"=w382) -> ("Module Admin out"=w381:refnum<class "Delacor_lib_QMH_Cloneable Module Admin.lvclass">)  [unwired: 9 in, 1 out]
      n159 = property class="Mod Admin"(reference=w381) -> ("Accessors:Module ID"=w380:i32)  [unwired: 1 in, 2 out]
      n160 = call "Module Name--constant.vi"("Module ID"=w380) -> ("Module Name"=w385:string)  [unwired: 10 in]
      n161 = call "Remove.vi"("Module ID"=w380) -> ()  [unwired: 9 in, 2 out]
      n162 = Format Into String(format string="An error occurred during initialization. %s is no longer running.", w385) -> (resulting string=w383:string)  [unwired: 2 in, 1 out]
      n163 = call "Error Reported.vi"("Additional Information"=w383, "Error"=w387, "Module ID"=w380) -> ()  [unwired: 8 in, 1 out]
    }
  }
  n164 = Merge Errors(w4, w34, w33, w12) -> (w35:errorcluster)
  n165 = call "Close Module.vi"("error in (no error)"=w35, "Wait for stop?"=w19, "Module Admin in"=w21) -> ("error out"=w31:errorcluster, "External Launch"=w18:bool, "Module Admin out"=w20:refnum<class "Delacor_lib_QMH_Cloneable Module Admin.lvclass">)  [unwired: 6 in]
  n166 = Unregister For Events(event registration refnum=w26, error in=w31) -> (error out=w30:errorcluster)
  n167 = Unregister For Events(event registration refnum=w2, error in=w30) -> (error out=w15:errorcluster)
  n168 = Unregister For Events(event registration refnum=w1, error in=w15) -> (error out=w3:errorcluster)
  "error out" <- w3
  n169 = local write "Module Admin"(w20) -> ()
  n170 = case "External Launch?" shown="True" w18 {
    tunnel: w3 -> [_ w388]
    frame False {
    }
    frame True {
      n171 = case shown="No Error" w388 {
        frame No Error {
          n172 = invoke class="VI" method="FP.Close"() -> ()  [unwired: 3 in, 3 out]
        }
        frame Error {
          n173 = invoke class="VI" method="FP.Open"("Activate"=TRUE ("Activate?")) -> ()  [unwired: 4 in, 5 out]
        }
      }
    }
  }
